vi "Set sweep parameters.vi"(5 "VDI config constants":T2, 9 "Sweep parameters":T4 {"Sweep down\ntime [ms]" min=0.0 max=250.0; "End [GHz]" min=8.0 max=20.0; "Intermidiate [MHz]" min=0.0 max=2500.0; "Start [GHz]" min=8.0 max=20.0}) -> (4 "data out1":u8[][](array[numeric]), 6 "data out 2":u8[][](array[numeric]), 8 "Freq limit reached":bool, 10 "Error1":bool, 15 "Error2":bool)   [LabVIEW 2021, in "THz source modeule.lvlib"]
uses:
  THz source modeule.lvlib
  ctl/THz sweep parameters.ctl
  ctl/VDI config constants.ctl
  ctl/Synth configs.ctl
panel:
  out "Folower Actual settings":T1 {"CWFreq(GHz)" format="%#_12g"; "RiseStepDwellTime(uS)" format="%#_12g"; "FallStepDwellTime(uS)" format="%#_12g"; "RiseTime(mS)" format="%#_14g"; "FallTime(mS)" format="%#_14g"; "StartFreq(GHz)" format="%#_12g"; "StopFreq(GHz)" format="%#_12g"; "RiseStepSize(Hz)" format="%#_12g"; "FallStepSize(Hz)" format="%#_12g"; "Rise#Steps" format="%#_12g"; "Fall#Steps" format="%#_12g"}
  out "Actual settings":T1 {"CWFreq(GHz)" format="%#_12g"; "RiseStepDwellTime(uS)" format="%#_12g"; "FallStepDwellTime(uS)" format="%#_12g"; "RiseTime(mS)" format="%#_14g"; "FallTime(mS)" format="%#_14g"; "StartFreq(GHz)" format="%#_12g"; "StopFreq(GHz)" format="%#_12g"; "RiseStepSize(Hz)" format="%#_12g"; "FallStepSize(Hz)" format="%#_12g"; "Rise#Steps" format="%#_12g"; "Fall#Steps" format="%#_12g"}
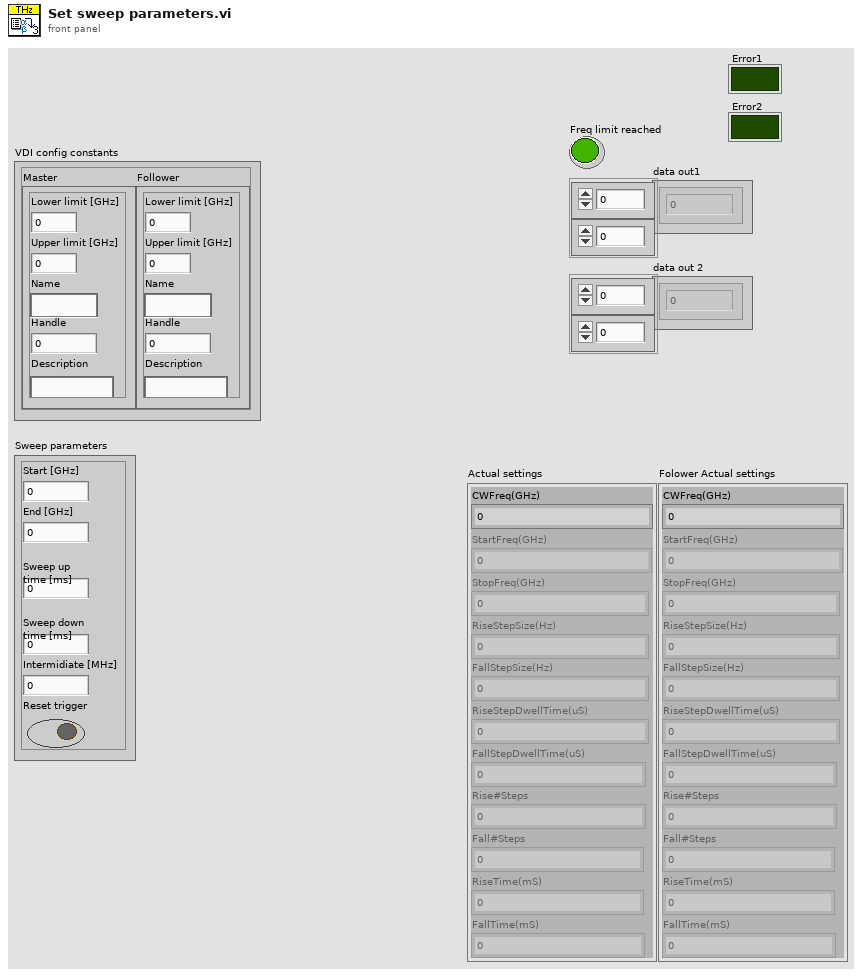
[diagram p1: front panel]
types:
  T1 = cluster{"CWFreq(GHz)":dbl, "StartFreq(GHz)":dbl, "StopFreq(GHz)":dbl, "RiseStepSize(Hz)":dbl, "FallStepSize(Hz)":dbl, "RiseStepDwellTime(uS)":dbl, "FallStepDwellTime(uS)":dbl, "Rise#Steps":dbl, "Fall#Steps":dbl, "RiseTime(mS)":dbl, "FallTime(mS)":dbl}
  T2 = typedef "VDI config constants.ctl" = cluster{"Master":T3, "Follower":T3}
  T3 = typedef "THz source modeule.lvlib/Synth configs.ctl" = cluster{"Lower limit [GHz]":dbl, "Upper limit [GHz]":dbl, "Name":string, "Handle":u32, "Description":string}
  T4 = typedef "THz source modeule.lvlib/THz sweep parameters.ctl" = cluster{"Start [GHz]":dbl, "End [GHz] ":dbl, "Sweep up\ntime [ms]":dbl, "Sweep down\ntime [ms]":dbl, "Intermidiate [MHz]":dbl, "Reset trigger":bool}
  T5 = cluster{"Numeric Control":dbl, "Numeric Control":dbl, i32, i32, i32, i32, "RiseFall Dwell Low":bool, "RiseFall Dwell High":bool, "Pause Sweep":bool, "Swep Direction":bool}
  T6 = cluster{"Lowest Sweep Frequency(GHz)":dbl, "Highest Sweep Frequency(GHz)":dbl, "Rising Step Size(GHz)":dbl, "Falling Step Size(GHz)":dbl, "Rising Step Time(uS)":dbl, "Falling Step Time(uS)":dbl, "Dwell Low":bool, "Dwell High":bool, "Sweep Pause":bool, "Sweep Direction":bool}
  T7 = cluster{"Upper limit [GHz]":dbl, "Upper limit [GHz]":dbl, i32, i32, i32, i32, bool, bool, bool, bool}
  T8 = cluster{"Upper limit [GHz]":dbl, "Upper limit [GHz]":dbl, i32, i32, i32, i32, bool, bool, bool, bool}[]
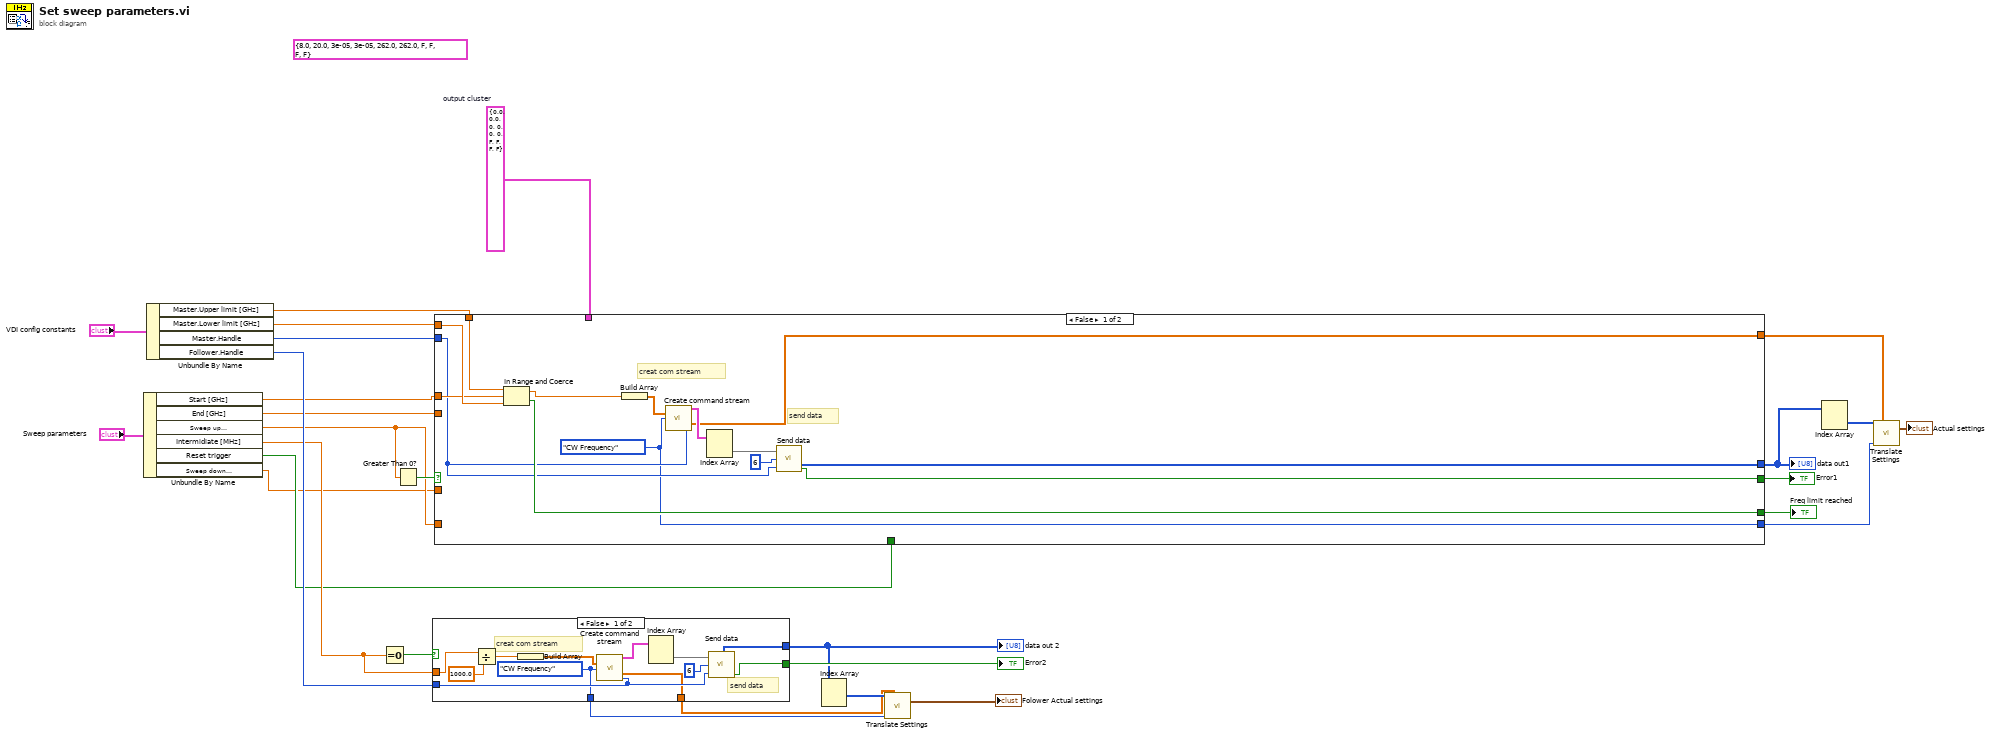
[diagram p0: block diagram]
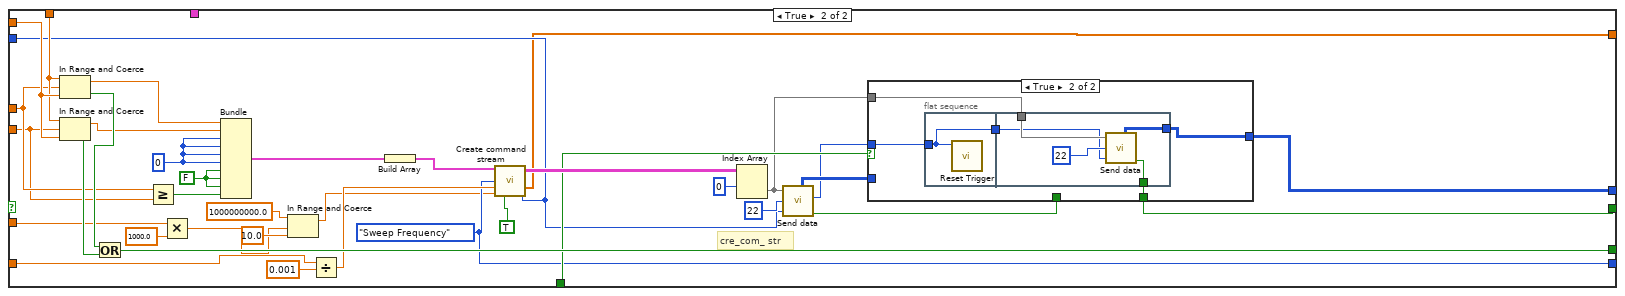
[diagram p3: hidden frame]
diagram:
  w14 = T5 {"Numeric Control"=0.0, "Numeric Control"=0.0, 0, 0, 0, 0, "RiseFall Dwell Low"=FALSE, "RiseFall Dwell High"=FALSE, "Pause Sweep"=FALSE, "Swep Direction"=FALSE}  # output cluster
  (unwired) T6 {"Lowest Sweep Frequency(GHz)"=8.0, "Highest Sweep Frequency(GHz)"=20.0, "Rising Step Size(GHz)"=3e-05, "Falling Step Size(GHz)"=3e-05, "Rising Step Time(uS)"=262.0, "Falling Step Time(uS)"=262.0, "Dwell Low"=FALSE, "Dwell High"=FALSE, "Sweep Pause"=FALSE, "Sweep Direction"=FALSE} ("Sweep Parameters")
  n1 = Unbundle By Name("Sweep parameters") -> ("Start [GHz]"=w18:dbl, "End [GHz]"=w21:dbl, "Sweep up\ntime [ms]"=w16:dbl, "Intermidiate [MHz]"=w26:dbl, "Reset trigger"=w13:bool, "Sweep down\ntime [ms]"=w6:dbl)
  n2 = Unbundle By Name("VDI config constants") -> ("Master.Upper limit [GHz]"=w22:dbl, "Master.Lower limit [GHz]"=w20:dbl, "Master.Handle"=w12:u32, "Follower.Handle"=w27:u32)
  n3 = Equal To 0?(x=w26) -> (x = 0?=w25:bool)
  n4 = Greater Than 0?(x=w16) -> (x > 0?=w17:bool)
  n5 = case shown="False" w25 {
    tunnel: w27 -> [w35 _]
    tunnel: w26 -> [w40 _]
    tunnel: [w34 _] -> w28
    tunnel: [w33 _] -> w5
    tunnel: [w30 _] -> w3
    tunnel: [w29 _] -> w2
    frame False {
      w29 = enum16{"CW Frequency", "Sweep Frequency"}."CW Frequency" ("Command mode")
      # "send data"
      # "creat com stream"
      n6 = Divide(x=w40, y=1000.0) -> (x/y=w32:dbl)
      n7 = Build Array(w32) -> (w38:dbl[])
      n8 = call <instrlib>:"Create command stream.vi"("CWfreq array(GHz)"=w38, "Command mode"=w29, "Handle"=w35) -> ("Data packets"=w39:cluster{"Write Data":u8[]}[][], "Output step time(uS)"=w30:dbl[])  [unwired: 11 in]
      n9 = Index Array(array=w39) -> (element=w37:cluster{"Write Data":u8[]}[])  [unwired: 2 in]
      n10 = call <instrlib>:"Send data.vi"("Data packets"=w37, "bytes to read"=6 ("index"), "Handle"=w35) -> ("data out"=w33:u8[][], "Error"=w34:bool)  [unwired: 3 in, 3 out]
    }
    frame True {
      # "No following synth"
    }
  }
  "Error2" <- w28
  "data out 2" <- w5
  n11 = case shown="False" w17 {
    tunnel: w18 -> [w52 w73]
    tunnel: w20 -> [w53 w91]
    tunnel: w21 -> [_ w72]
    tunnel: w22 -> [w54 w90]
    tunnel: w14 -> [_ _]
    tunnel: w16 -> [_ w70]
    tunnel: w12 -> [w44 w69]
    tunnel: [w45 w65] -> w23
    tunnel: [w50 w81] -> w15
    tunnel: [w46 w64] -> w11
    tunnel: w13 -> [_ w74]
    tunnel: [w42 w62] -> w9
    tunnel: [w41 w61] -> w8
    tunnel: w6 -> [_ w59]
    frame False {
      w41 = enum16{"CW Frequency", "Sweep Frequency"}."CW Frequency" ("Command mode")
      # "send data"
      # "creat com stream"
      n12 = In Range and Coerce(upper limit=w54, x=w52, lower limit=w53) -> (coerced(x)=w51:dbl, In Range?=w50:bool)
      n13 = Build Array(w51) -> (w43:dbl[])
      n14 = call <instrlib>:"Create command stream.vi"("CWfreq array(GHz)"=w43, "Command mode"=w41, "Handle"=w44) -> ("Data packets"=w49:cluster{"Write Data":u8[]}[][], "Output step time(uS)"=w42:dbl[])  [unwired: 11 in]
      n15 = Index Array(array=w49) -> (element=w48:cluster{"Write Data":u8[]}[])  [unwired: 2 in]
      n16 = call <instrlib>:"Send data.vi"("Data packets"=w48, "bytes to read"=6 ("index"), "Handle"=w44) -> ("data out"=w46:u8[][], "Error"=w45:bool)  [unwired: 3 in, 3 out]
    }
    frame True {
      w61 = enum16{"CW Frequency", "Sweep Frequency"}."Sweep Frequency" ("Command mode")
      w86 = FALSE
      w87 = 0
      # "cre_com_ str"
      n17 = In Range and Coerce(upper limit=w90, x=w73, lower limit=w91) -> (coerced(x)=w84:dbl, In Range?=w89:bool)
      n18 = In Range and Coerce(upper limit=w90, x=w72, lower limit=w91) -> (coerced(x)=w83:dbl, In Range?=w88:bool)
      n19 = Or(x=w89, y=w88) -> (x .or. y?=w81:bool)
      n20 = Greater Or Equal?(x=w73, y=w72) -> (x >= y?=w71:bool)
      n21 = Multiply(x=w59, y=1000.0 ("Sweep down\ntime [ms]")) -> (x*y=w56:dbl)
      n22 = Bundle("Upper limit [GHz]"=w84, "Upper limit [GHz]"=w83, w87, w87, w87, w87, w86, w86, w86, w71) -> (w85:T7)  [unwired: 1 in]
      n23 = In Range and Coerce(upper limit=1000000000.0, x=w56, lower limit=10.0) -> (coerced(x)=w60:dbl)  [unwired: 1 out]
      n24 = Divide(x=w70, y=0.001) -> (x/y=w78:dbl)
      n25 = Build Array(w85) -> (w80:T8)
      n26 = call <instrlib>:"Create command stream.vi"("Sweep Parameters"=w80, "Command mode"=w61, "Rising Sweep Time(uS)"=w78, "Falling Sweep Time(uS)"=w60, "Calculate step size,time"=TRUE, "Handle"=w69) -> ("Data packets"=w79:cluster{"Write Data":u8[]}[][], "Output step time(uS)"=w62:dbl[])  [unwired: 8 in]
      n27 = Index Array(array=w79, index (row)=0) -> (element=w67:cluster{"Write Data":u8[]}[])  [unwired: 1 in]
      n28 = call <instrlib>:"Send data.vi"("Data packets"=w67, "bytes to read"=u32 22, "Handle"=w69) -> ("data out"=w68:u8[][], "Handle out"=w66:u32, "Error"=w63:bool)  [unwired: 3 in, 2 out]
      n29 = case shown="True" w74 {
        tunnel: w66 -> [_ w98]
        tunnel: w68 -> [w93 _]
        tunnel: w67 -> [_ w97]
        tunnel: [w92 w96] -> w65
        tunnel: [w93 w95] -> w64
        tunnel: w63 -> [w92 _]
        frame False {
        }
        frame True {
          n30 = flat-sequence {
            tunnel: w98 -> [w99]
            tunnel: [w99] -> w94
            tunnel: w97 -> [w104]
            tunnel: [w102] -> w96
            tunnel: [w101] -> w95
            tunnel: w94 -> [w100]
            frame #0 {
              n31 = call <instrlib>:"Reset Trigger.vi"("Handle"=w99) -> ()  [unwired: 11 in]
            }
            frame #1 {
              n32 = call <instrlib>:"Send data.vi"("Data packets"=w104, "bytes to read"=u32 22, "Handle"=w100) -> ("data out"=w101:u8[][], "Error"=w102:bool)  [unwired: 3 in, 3 out]
            }
          }
        }
      }
    }
  }
  "Error1" <- w23
  "Freq limit reached" <- w15
  "data out1" <- w11
  n33 = Index Array(array=w5) -> (element=w4:u8[])  [unwired: 2 in]
  n34 = call "Translate Settings.vi"("data"=w4, "Step time(uS)"=w3, "Command mode"=w2) -> ("Actual settings"=→"Folower Actual settings":T1)  [unwired: 12 in]
  n35 = Index Array(array=w11) -> (element=w10:u8[])  [unwired: 2 in]
  n36 = call "Translate Settings.vi"("data"=w10, "Step time(uS)"=w9, "Command mode"=w8) -> ("Actual settings"=→"Actual settings":T1)  [unwired: 12 in]
